vi "2013_01_03 Each Motor.vi"(6 "Temp On":dbl=1.0, 8 "Motor #":i32=1, 9 "data":waveform(dbl)[](array[waveform]), 10 "File Path":path=path "Durability/.lvm", 11 "Motor Typedef":T1 {"Elec Power In (W)" format="%.3g"; "Efficiency" format="%#_3g%%"; "Mech Pwr Out (W)" format="%.3g"; "Torque (mNm)" format="%.3g"; "Elapsed Time" format="%<%H:%M:%S>t"; "Supply (V)" format="%.2f"; "RPM" scale=0.0..40000.0 scale format="%#_4p"}) -> (0 "Final Out":dynamicdata(graph), 3 "Motor Typedef Out":T1={"Enabled"=FALSE, "Fail"=FALSE, "RPM"=0.0, "Motor"=enum."Maxon EC6 6V", "ESC"=enum."Phoenix", "Supply (V)"=0.0, "Test ID and Serial #"="", "Comments"="", "Elapsed Time"=0.0, "Counter"=0.0, "Torque (mNm)"=0.0, "Mech Pwr Out (W)"=0.0, "Efficiency"=0.0, "Elec Power In (W)"=0.0} {"Elec Power In (W)" format="%.3g"; "Efficiency" format="%#_3g%%"; "Mech Pwr Out (W)" format="%.3g"; "Torque (mNm)" format="%.3g"; "Elapsed Time" format="%<%H:%M:%S>t"; "Supply (V)" format="%.2f"; "RPM" scale=0.0..40000.0 scale format="%#_4p"})   [LabVIEW 2012]
uses:
  MotorTypeDef.ctl
  <vilib>/express/express shared/transition.llb/Dynamic To Waveform Array.vi
  <vilib>/express/express signal manip/GetorSetDDTAttributes/Set DDT Attributes/SetT0.vi
  <vilib>/express/express shared/transition.llb/Waveform Array To Dynamic.vi
  <vilib>/express/express signal manip/GetorSetDDTAttributes/Set DDT Attributes/Set DDT Properties.xnode
panel:
  in  "error in (no error)":errorcluster
  out "error out":errorcluster
  out "Saving Data":bool
  # "Enable"
  # "Fail"
  # "Enable"
  # "Fail"
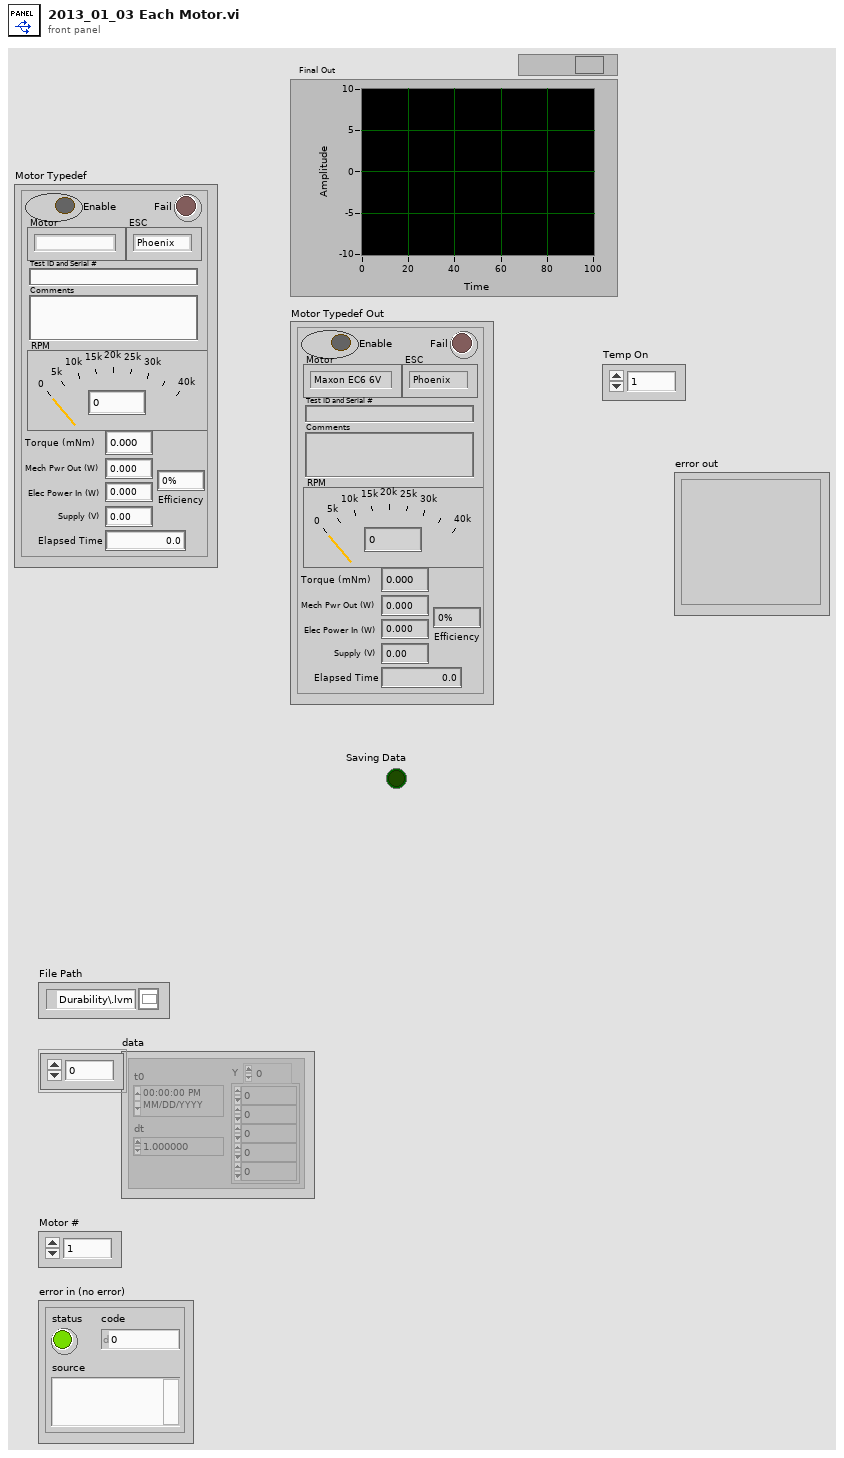
[diagram p1: front panel]
types:
  T1 = typedef "MotorTypeDef.ctl" = cluster{"Enabled":bool, "Fail":bool, "RPM":dbl, "Motor":enum16{"", "Maxon EC6 6V", "Maxon EC4 6V", "FH 0620 6V", "FH 0620 12V"}, "ESC":enum16{"Phoenix", "Maxon", "FH 1801"}, "Supply (V)":dbl, "Test ID and Serial #":string, "Comments":string, "Elapsed Time":dbl, "Counter":dbl, "Torque (mNm)":dbl, "Mech Pwr Out (W)":dbl, "Efficiency":dbl, "Elec Power In (W)":dbl}
  T2 = enum16{"", "Maxon EC6 6V", "Maxon EC4 6V", "FH 0620 6V", "FH 0620 12V"}
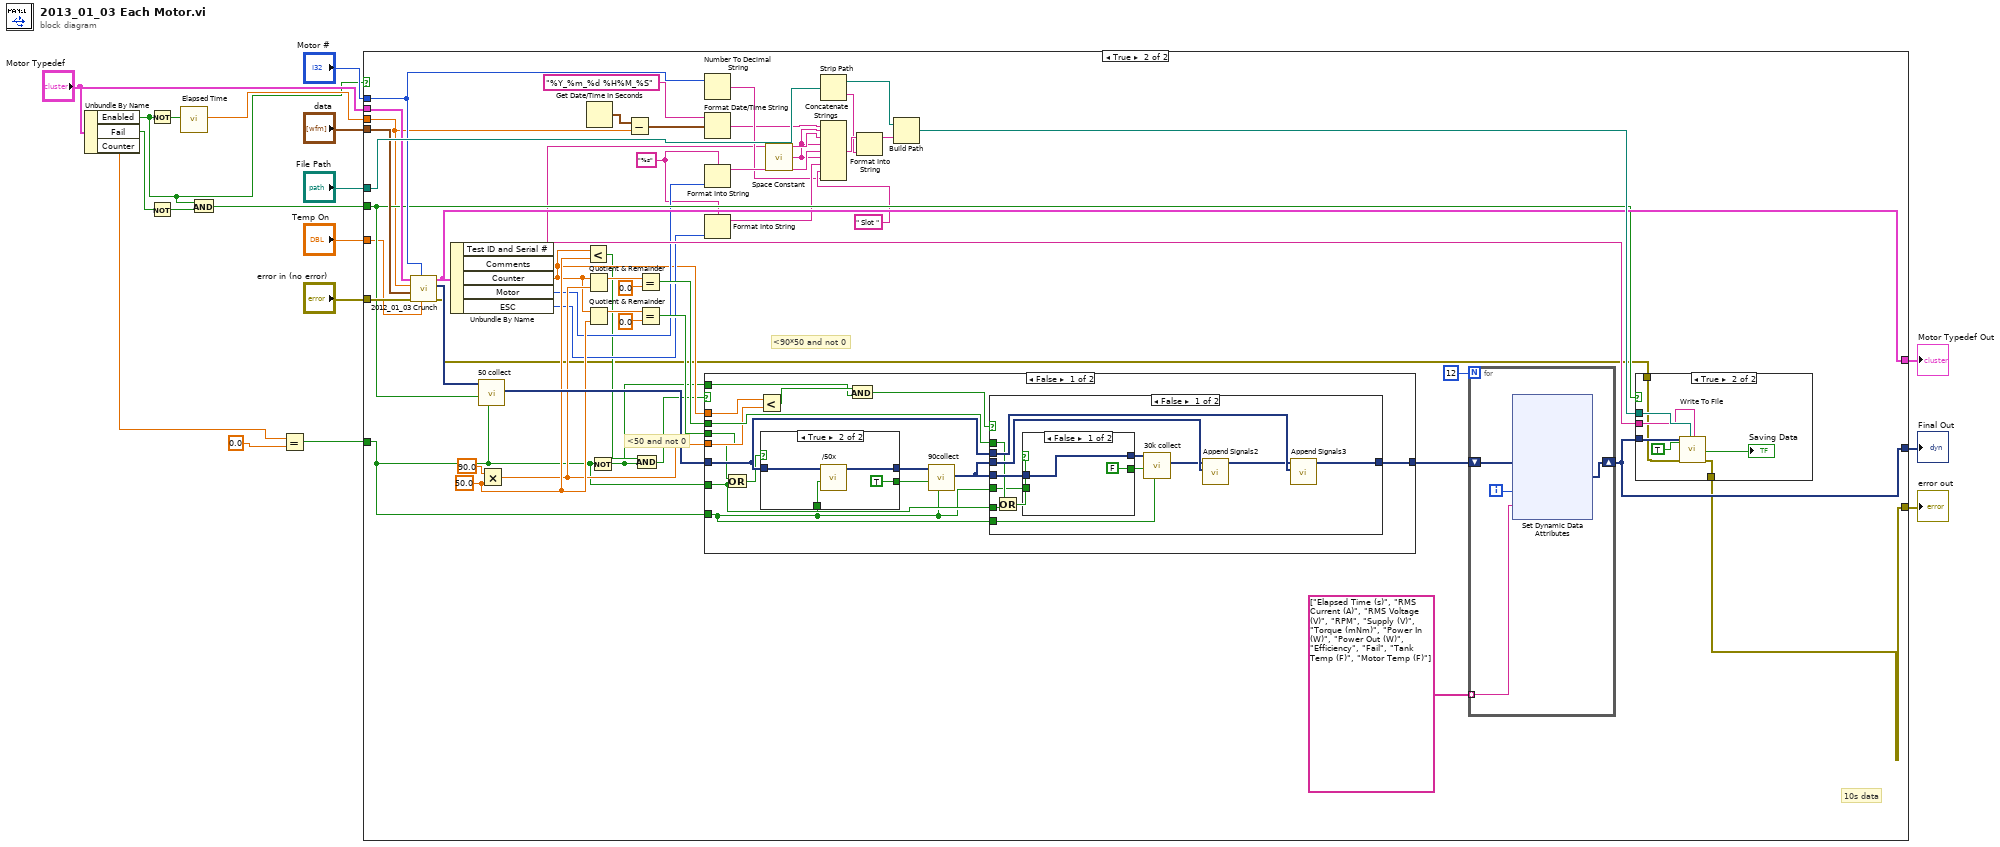
[diagram p0: block diagram]
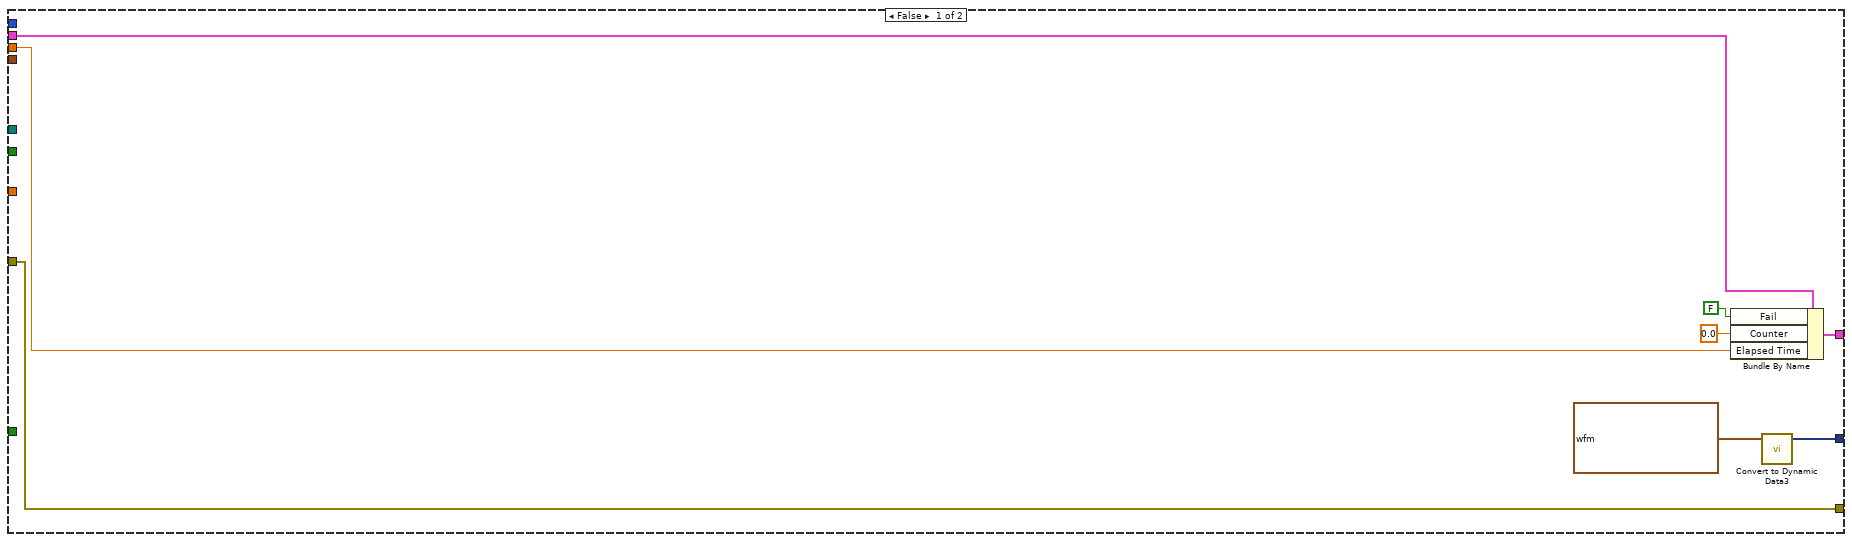
[diagram p2: hidden frame]
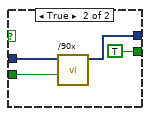
[diagram p3: hidden frame]
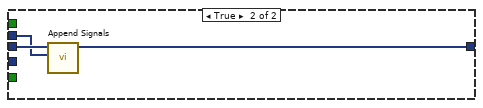
[diagram p4: hidden frame]
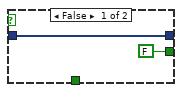
[diagram p5: hidden frame]
diagram:
  n1 = Unbundle By Name("Motor Typedef") -> ("Enabled"=w6:bool, "Fail"=w8:bool, "Counter"=w1:dbl)
  n2 = Not(x=w6) -> (.not. x?=w14:bool)
  n3 = Not(x=w8) -> (.not. x?=w7:bool)
  n4 = call "Elapsed Time"("Reset"=w14) -> ("Elapsed Time (s)"=w12:dbl)  [unwired: 11 in, 7 out]
  n5 = And(x=w6, y=w7) -> (x .and. y?=w5:bool)
  n6 = Equal?(x=w1, y=0.0) -> (x = y?=w3:bool)
  n7 = case shown="True" w6 {
    tunnel: "File Path" -> [_ w76]
    tunnel: [w23 w28] -> w17
    tunnel: "error in (no error)" -> [w23 w75]
    tunnel: "data" -> [_ w74]
    tunnel: [w20 w51] -> w13
    tunnel: w12 -> [w25 w47]
    tunnel: "Motor #" -> [_ w67]
    tunnel: "Motor Typedef" -> [w26 w66]
    tunnel: [w24 w55] -> w9
    tunnel: w5 -> [_ w49]
    tunnel: "Temp On" -> [_ w44]
    tunnel: w3 -> [_ w29]
    frame False {
      n8 = Bundle By Name(cluster=w26, "Fail"=FALSE, "Counter"=0.0, "Elapsed Time"=w25) -> (w24:T1)
      n9 = call "Convert to Dynamic Data3"("Waveform"=waveform(dbl) {"t0"=timestamp(0 s since 1904-01-01), "dt"=1.0, "Y"=[]}) -> ("Dynamic Data Type"=w20:dynamicdata)  [unwired: 3 in]
    }
    frame True {
      w40 = "%s" ("format string")
      w59 = 50.0 ("y")
      # "<90*50 and not 0"
      # "<50 and not 0"
      # "10s data"
      n10 = call "2012_01_03 Crunch.vi"("Temp On"=w44, "Motor #"=w67, "error in (no error)"=w75, "data"=w74, "Elapsed Time (s)"=w47, "Motor In"=w66) -> ("error out"=w27:errorcluster, "Dynamic Data Type"=w62:dynamicdata, "Motor Out"=w55:T1)  [unwired: 3 in]
      n11 = Unbundle By Name(w55) -> ("Test ID and Serial #"=w36:string, "Comments"=w68:string, "Counter"=w33:dbl, "Motor"=w43:T2, "ESC"=w39:enum16{"Phoenix", "Maxon", "FH 1801"})
      n12 = call "50 collect"("Reset"=w29, "Enable"=w49, "Signals"=w62) -> ("Collected Signals"=w60:dynamicdata)  [unwired: 7 in, 1 out]
      n13 = Multiply(x=90.0 ("y"), y=w59) -> (x*y=w54:dbl)
      n14 = Less?(x=w33, y=w59) -> (x < y?=w31:bool)
      n15 = Quotient & Remainder(x=w33, y=w54) -> (x-y*floor(x/y)=w58:dbl)  [unwired: 1 out]
      n16 = Quotient & Remainder(x=w33, y=w59) -> (x-y*floor(x/y)=w64:dbl)  [unwired: 1 out]
      n17 = Get Date/Time In Seconds() -> (seconds since 1Jan1904=w48:timestamp)
      n18 = Not(x=w29) -> (.not. x?=w30:bool)
      n19 = Subtract(x=w48, y=w47) -> (x-y=w46:timestamp)
      n20 = And(x=w31, y=w30) -> (x .and. y?=w32:bool)
      n21 = Equal?(x=w58, y=0.0) -> (x = y?=w56:bool)
      n22 = Equal?(x=w64, y=0.0) -> (x = y?=w61:bool)
      n23 = Number To Decimal String(number=w67) -> (decimal integer string=w37:string)  [unwired: 1 in]
      n24 = Format Date/Time String(time format string (%c)="%Y_%m_%d %H%M_%S", seconds (now)=w46) -> (date/time string=w34:string)  [unwired: 1 in]
      n25 = Format Into String(format string=w40, w43) -> (resulting string=w42:string)  [unwired: 2 in, 1 out]
      n26 = Format Into String(format string=w40, w39) -> (resulting string=w41:string)  [unwired: 2 in, 1 out]
      n27 = case shown="False" w32 {
        tunnel: w61 -> [w97 _]
        tunnel: w60 -> [w102 w137]
        tunnel: [w101 w137] -> w50
        tunnel: w56 -> [w106 _]
        tunnel: w33 -> [w105 _]
        tunnel: w54 -> [w104 _]
        tunnel: w29 -> [w94 _]
        tunnel: w30 -> [w99 _]
        tunnel: w29 -> [w95 _]
        frame False {
          n28 = Or(x=w97, y=w95) -> (x .or. y?=w96:bool)
          n29 = Less?(x=w105, y=w104) -> (x < y?=w100:bool)
          n30 = case shown="True" w96 {
            tunnel: w102 -> [w132 w136]
            tunnel: [w132 w135] -> w108
            tunnel: [FALSE ("x = y?") TRUE ("x = y?")] -> w107
            tunnel: w94 -> [_ w133]
            frame False {
            }
            frame True {
              n31 = call "/50x"("Reset"=w133, "Signals"=w136) -> ("Mean"=w135:dynamicdata)  [unwired: 7 in, 2 out]
            }
          }
          n32 = And(x=w100, y=w99) -> (x .and. y?=w98:bool)
          n33 = call "90collect"("Reset"=w94, "Enable"=w107, "Signals"=w108) -> ("Collected Signals"=w103:dynamicdata)  [unwired: 7 in, 1 out]
          n34 = case shown="False" w98 {
            tunnel: w103 -> [w119 _]
            tunnel: w106 -> [w112 _]
            tunnel: w103 -> [w116 w130]
            tunnel: w102 -> [w118 w129]
            tunnel: [w114 w128] -> w101
            tunnel: w94 -> [w113 _]
            tunnel: w95 -> [w111 _]
            tunnel: w94 -> [w109 _]
            frame False {
              n35 = Or(x=w112, y=w111) -> (x .or. y?=w110:bool)
              n36 = case shown="False" w110 {
                tunnel: w119 -> [w123 w127]
                tunnel: [w123 w126] -> w121
                tunnel: [FALSE ("x = y?") TRUE ("x = y?")] -> w120
                tunnel: w109 -> [_ w124]
                frame False {
                }
                frame True {
                  n37 = call "/90x"("Reset"=w124, "Signals"=w127) -> ("Mean"=w126:dynamicdata)  [unwired: 7 in, 2 out]
                }
              }
              n38 = call "30k collect"("Reset"=w113, "Enable"=w120, "Signals"=w121) -> ("Collected Signals"=w115:dynamicdata)  [unwired: 7 in, 1 out]
              n39 = call "Append Signals2"("Input Signal B"=w116, "Input Signal A"=w115) -> ("Appended Signals"=w117:dynamicdata)  [unwired: 8 in, 1 out]
              n40 = call "Append Signals3"("Input Signal B"=w118, "Input Signal A"=w117) -> ("Appended Signals"=w114:dynamicdata)  [unwired: 8 in, 1 out]
            }
            frame True {
              n41 = call "Append Signals"("Input Signal B"=w129, "Input Signal A"=w130) -> ("Appended Signals"=w128:dynamicdata)  [unwired: 8 in, 1 out]
            }
          }
        }
        frame True {
        }
      }
      n42 = call <vilib>:"Space Constant.vi"() -> ("String"=w35:string)
      n43 = Strip Path(path=w76) -> (stripped path=w70:path, name=w71:string)
      n44 = Concatenate Strings(w34, w35, w36, w35, w42, w35, w41, " Slot " ("string"), w37) -> (w72:string)
      n45 = Format Into String(initial string=w72, w71) -> (resulting string=w69:string)  [unwired: 2 in, 1 out]
      n46 = Build Path(base path=w70, name or relative path=w69) -> (appended path=w73:path)
      n47 = for {
        N: 12 -> [_]
        tunnel: string[] ["Elapsed Time (s)", "RMS Current (A)", "RMS Voltage (V)", "RPM", "Supply (V)", "Torque (mNm)", "Power In (W)", "Power Out (W)", "Efficiency", "Fail", "Tank Temp (F)", "Motor Temp (F)"] ("appended array") -> [w78] mode=indexing
        shift-right: [w79] -> w51
        shift-left: w50 -> [w77]
        i -> [w80]
        n48 = xnode "Set Dynamic Data Attributes"("Signals In"=w77, "Signal Index"=w80, "Signal Name"=w78) -> ("Signals Out"=w79:dynamicdata)  [unwired: 1 in, 1 out]
      }
      n49 = case shown="True" w49 {
        tunnel: w51 -> [_ w145]
        tunnel: w73 -> [_ w144]
        tunnel: w68 -> [_ w141]
        tunnel: [w138 w140] -> w28
        tunnel: w27 -> [w138 w139]
        frame False {
        }
        frame True {
          n50 = call "Write To File"("Signals"=w145, "Reset"=TRUE, "error in (no error)"=w139, "Filename"=w144, "Comment"=w141) -> ("Saving Data"=→"Saving Data":bool, "error out"=w140:errorcluster)  [unwired: 12 in, 1 out]
        }
      }
    }
  }
  "error out" <- w17
  "Final Out" <- w13
  "Motor Typedef Out" <- w9
